vi "test random.vi"() -> ()   [LabVIEW 2018, in "LV-0mq-Julia_roundtrip-lib.lvlib"]
uses:
  LV-0mq-Julia_roundtrip-lib.lvlib
  8ff801c8-b98c-4af1-845c-0726e8db660c.vi
panel:
  out "Bool out":bool=TRUE
  out "complex out":cdb
  out "float out":dbl
  in  "type in":bool
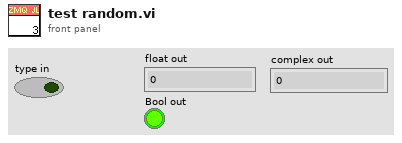
[diagram p1: front panel]
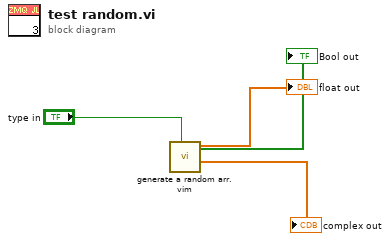
[diagram p0: block diagram]
diagram:
  n1 = call "generate a random arr.vim"("type in"="type in") -> ("float out"=→"float out":dbl[], "complex out"=→"complex out":cdb[], "Bool out"=→"Bool out":bool[])  [unwired: 6 in, 2 out]
